vi "inputPopup.vi"(10 "default text":string, 11 "Label.Text":string) -> (3 "value":string)   [LabVIEW 2013]
panel:
  in  "String":string caption="Enter new path:"
  in  "Cancel Button":bool
  in  "OK Button":bool
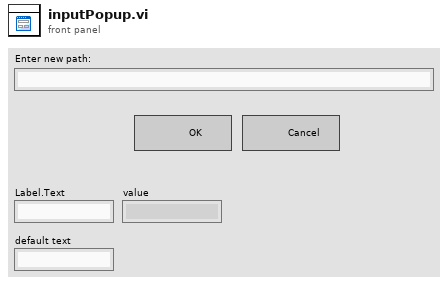
[diagram p1: front panel]
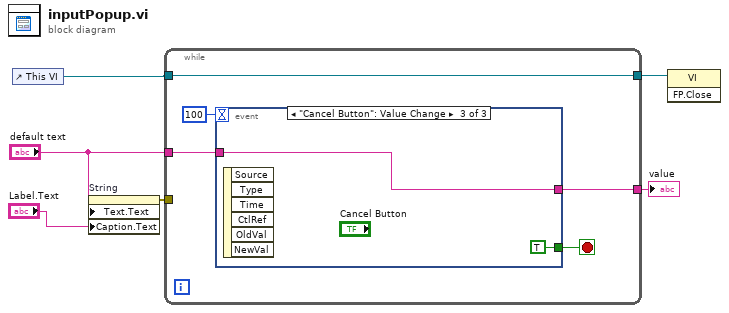
[diagram p0: block diagram]
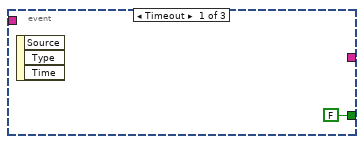
[diagram p2: hidden frame]
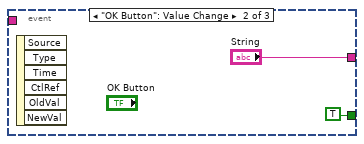
[diagram p3: hidden frame]
diagram:
  n1 = control-ref of="This VI"() -> (w1:refnum<vi>)
  n2 = property on="String" class="Str"("Text.Text"="default text", "Caption.Text"="Label.Text") -> (error out=w5:errorcluster)  [unwired: 2 in, 1 out]
  n3 = while {
    tunnel: [w10] -> w6
    tunnel: w5 -> [_]
    tunnel: "default text" -> [w9]
    tunnel: w1 -> [w7]
    tunnel: [w7] -> w2
    stop <- w11 stop-if-true
    n4 = event shown="[2] \"Cancel Button\": Value Change" {
      selector: _ -> [_ _ _]
      dyn-events: _ -> [_ _ _]
      timeout: 100 -> [_ _ _]
      tunnel: [FALSE TRUE TRUE] -> w11
      tunnel: [_ "String" w16] -> w10
      tunnel: w9 -> [_ _ w16]
      event Timeout {
        n5 = event-data() -> ()  [unwired: 1 in, 3 out]
      }
      event "OK Button": Value Change {
        n6 = event-data() -> ()  [unwired: 1 in, 6 out]
      }
      event "Cancel Button": Value Change {
        n7 = event-data() -> ()  [unwired: 1 in, 6 out]
      }
    }
  }
  "value" <- w6
  n8 = invoke class="VI" method="FP.Close"(reference=w2) -> ()  [unwired: 2 in, 3 out]
